vi "FPGA Wizard.vi"() -> ()   [LabVIEW 2015]
uses:
  Classes/Project/FPGA Settings.ctl
  Classes/Module/Module/Module Settings.ctl
  Classes/Signal/Signal/Signal Settings.ctl
  Classes/Project/Project.lvclass
  Classes/Module/Module/Module.lvclass
  Classes/Signal/Signal/Signal.lvclass
panel:
  out "FPGA Settings":T1[](array[typedef])
  out "error out":errorcluster
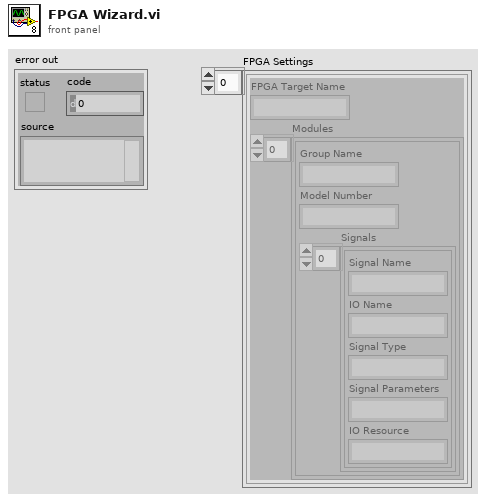
[diagram p1: front panel]
types:
  T1 = typedef "Project.lvclass/FPGA Settings.ctl" = cluster{"FPGA Target Name":string, "Modules":T2[]}
  T2 = typedef "Module.lvclass/Module Settings.ctl" = cluster{"Group Name":string, "Model Number":string, "Signals":T3[]}
  T3 = typedef "Signal.lvclass/Signal Settings.ctl" = cluster{"Signal Name":string, "IO Name":string, "Signal Type":string, "Signal Parameters":string, "IO Resource":string}
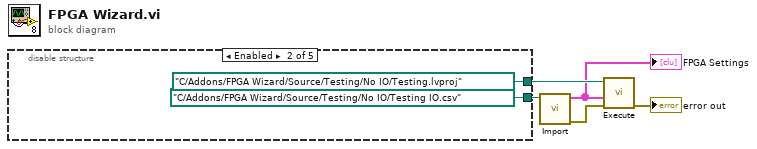
[diagram p0: block diagram]
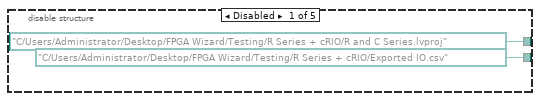
[diagram p2: hidden frame]
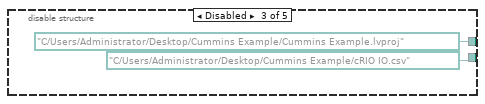
[diagram p3: hidden frame]
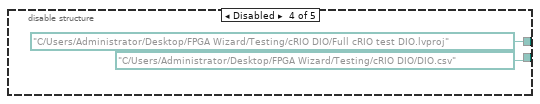
[diagram p4: hidden frame]
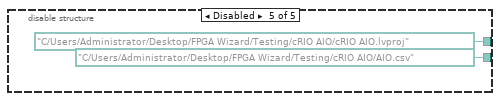
[diagram p5: hidden frame]
diagram:
  n1 = disable-structure shown="Enabled" {
    disable-tunnel: [path "C:/Users/Administrator/Desktop/FPGA Wizard/Testing/R Series + cRIO/R and C Series.lvproj" ("Project Path") path "C:/Addons/FPGA Wizard/Source/Testing/No IO/Testing.lvproj" ("Project Path") path "C:/Users/Administrator/Desktop/Cummins Example/Cummins Example.lvproj" ("Project Path") path "C:/Users/Administrator/Desktop/FPGA Wizard/Testing/cRIO DIO/Full cRIO test DIO.lvproj" ("Project Path") path "C:/Users/Administrator/Desktop/FPGA Wizard/Testing/cRIO AIO/cRIO AIO.lvproj" ("Project Path")] -> w5
    disable-tunnel: [path "C:/Users/Administrator/Desktop/FPGA Wizard/Testing/R Series + cRIO/Exported IO.csv" ("CSV Path") path "C:/Addons/FPGA Wizard/Source/Testing/No IO/Testing IO.csv" ("CSV Path") path "C:/Users/Administrator/Desktop/Cummins Example/cRIO IO.csv" ("CSV Path") path "C:/Users/Administrator/Desktop/FPGA Wizard/Testing/cRIO DIO/DIO.csv" ("CSV Path") path "C:/Users/Administrator/Desktop/FPGA Wizard/Testing/cRIO AIO/AIO.csv" ("CSV Path")] -> w1
    frame Disabled {
    }
    frame Enabled {
    }
    frame Disabled {
    }
    frame Disabled {
    }
    frame Disabled {
    }
  }
  n2 = call "Import.vi"("CSV Path"=w1) -> ("error out"=w3:errorcluster, "FPGA Settings"=w2:T1[])  [unwired: 9 in]
  "FPGA Settings" <- w2
  n3 = call "Execute.vi"("error in (no error)"=w3, "Targets"=w2, "Project Path"=w5) -> ("error out"=→"error out":errorcluster)  [unwired: 8 in]
